vi "LoadAutonomousPlays.vi"(8 "error in":errorcluster) -> (0 "error out":errorcluster)   [LabVIEW 2015]
uses:
  Play Info.ctl
  Autonomous Global.vi
  <vilib>/Rock Robotics/Network Tables/NT Write String Array.vi
panel:
  out "Array":T1[](array[typedef])
  out "filenames":string[](array[string])
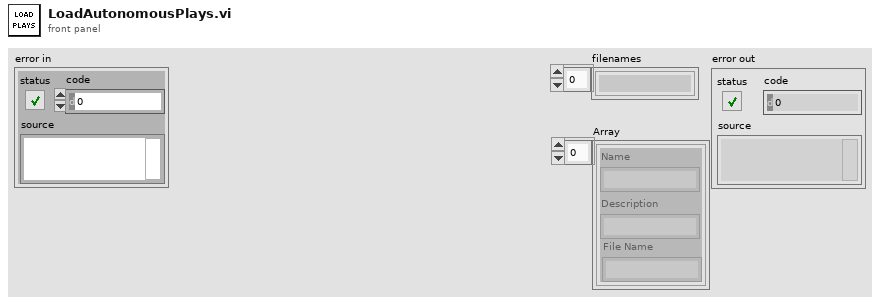
[diagram p1: front panel]
types:
  T1 = typedef "Play Info.ctl" = cluster{"Name":string, "Description":string, "File Name":string}
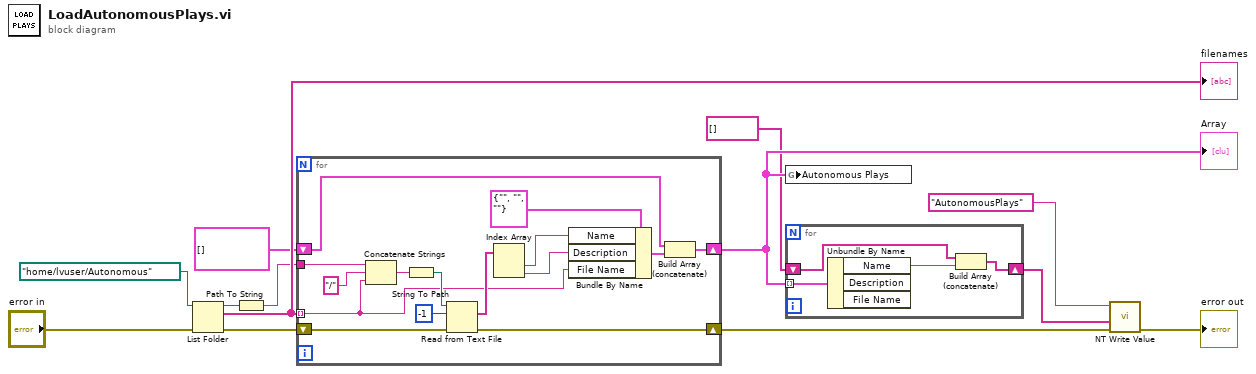
[diagram p0: block diagram]
diagram:
  n1 = List Folder(path=path "/home/lvuser/Autonomous", error in="error in") -> (path out=w9:path, filenames=w10:string[], error out=w11:errorcluster)  [unwired: 2 in, 1 out]
  "filenames" <- w10
  n2 = Path To String(path=w9) -> (string=w8:string)
  n3 = for {
    shift-right: [w27] -> w2
    shift-left: w11 -> [w28]
    tunnel: w10 -> [w14] mode=indexing
    tunnel: w8 -> [w25]
    shift-right: [w16] -> w6
    shift-left: T1[] [] -> [w15]
    n4 = Concatenate Strings(w25, "/" ("string"), w14) -> (w26:string)
    n5 = String To Path(string=w26) -> (path=w23:path)
    n6 = Read from Text File(file (use dialog)=w23, count=-1, error in=w28) -> (text=w21:string[], error out=w27:errorcluster)  [unwired: 1 in, 2 out]
    n7 = Index Array(array=w21) -> (element #1=w19:string, element #2=w18:string)  [unwired: 2 in]
    n8 = Bundle By Name(cluster=T1 {"Name"="", "Description"="", "File Name"=""} ("Play Info"), "Name"=w19, "Description"=w18, "File Name"=w14) -> (w17:T1)
    n9 = Build Array (concatenate)(w15, w17) -> (w16:T1[])
  }
  "Array" <- w6
  n10 = global write "Autonomous Global.vi" "Autonomous Plays"(w6) -> ()
  n11 = for {
    tunnel: w6 -> [w32] mode=indexing
    shift-right: [w30] -> w4
    shift-left: string[] [] -> [w29]
    n12 = Unbundle By Name(w32) -> ("Name"=w31:string)  [unwired: 2 out]
    n13 = Build Array (concatenate)(w29, w31) -> (w30:string[])
  }
  n14 = call-poly <vilib>:"NT Write Value.vi"("error in"=w2, "String Array"=w4, "Name"="AutonomousPlays") -> ("error out"=→"error out":errorcluster)  [unwired: 8 in]
